vi "Read wavelengths.vi"(8 "error in (no error)":errorcluster, 11 "DATA in":refnum<class "DATA.lvclass">) -> (0 "error out":errorcluster, 2 "wavelengths":dbl[](array[numeric]), 3 "DATA out":refnum<class "DATA.lvclass">)   [LabVIEW 2020, in "DATA.lvclass"]
uses:
  DATA.lvclass
  DATA.lvclass/DATA.ctl
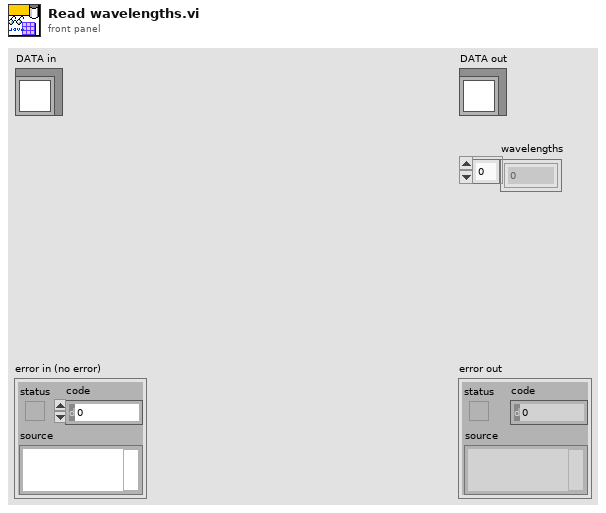
[diagram p1: front panel]
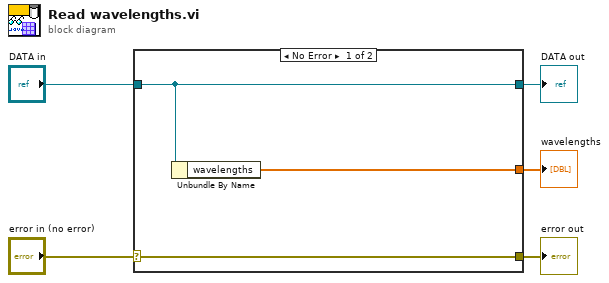
[diagram p0: block diagram]
diagram:
  n1 = case shown="No Error" "error in (no error)" {
    selector: "error in (no error)" -> [w8 w9]
    tunnel: [w8 w9] -> w4
    tunnel: [w7 w10] -> w2
    tunnel: "DATA in" -> [w7 w10]
    tunnel: [w6 _] -> w1
    frame No Error {
      n2 = Unbundle By Name(w7) -> ("wavelengths"=w6:dbl[])
    }
    frame Error {
    }
  }
  "error out" <- w4
  "DATA out" <- w2
  "wavelengths" <- w1
